vi "step5 TestIfUpperCrossAligned.vi"(8 "error in (no error)":errorcluster, 11 "cube in":T1) -> (0 "error out":errorcluster, 2 "upper cross aligned?":bool)   [LabVIEW 2011]
uses:
  Typedef/cube.ctl
  Typedef/face.ctl
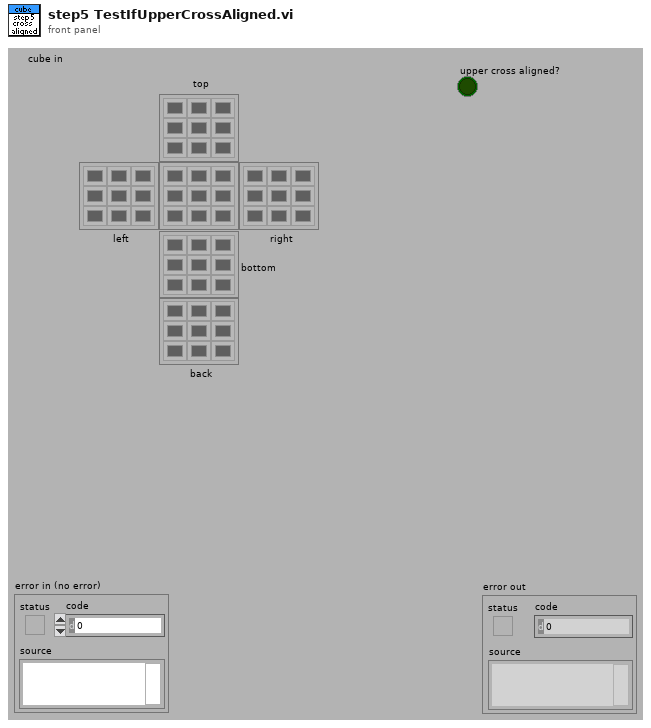
[diagram p1: front panel]
types:
  T1 = typedef "cube.ctl" = cluster{"top":T2, "left":T2, "right":T2, "bottom":T2, "back":T2, "front":T2}
  T2 = typedef "face.ctl" = u32[][]
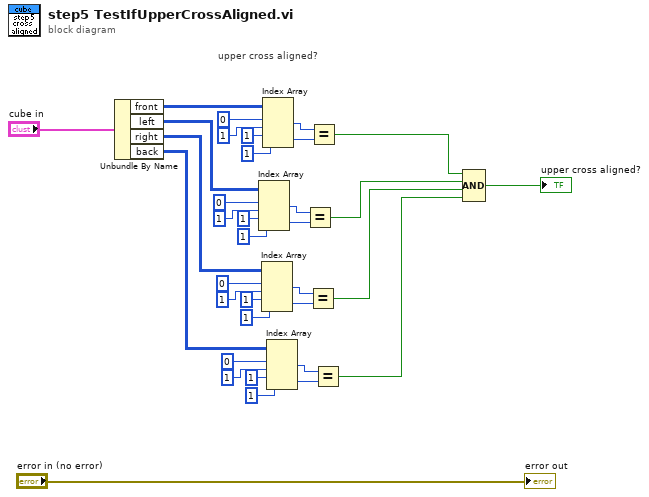
[diagram p0: block diagram]
diagram:
  # "upper cross aligned?"
  n1 = Unbundle By Name("cube in") -> ("front"=w31:T2, "left"=w18:T2, "right"=w11:T2, "back"=w4:T2)
  n2 = Index Array(array=w18, index (row) #1=0 ("index (row)"), index (col) #1=1 ("disabled index (col)"), index (row) #2=1 ("index (row)"), index (col) #2=1 ("disabled index (col)")) -> (element #1=w23:u32, element #2=w24:u32)
  n3 = Index Array(array=w11, index (row) #1=0 ("index (row)"), index (col) #1=1 ("disabled index (col)"), index (row) #2=1 ("index (row)"), index (col) #2=1 ("disabled index (col)")) -> (element #1=w13:u32, element #2=w12:u32)
  n4 = Index Array(array=w31, index (row) #1=0 ("index (row)"), index (col) #1=1 ("disabled index (col)"), index (row) #2=1 ("index (row)"), index (col) #2=1 ("disabled index (col)")) -> (element #1=w26:u32, element #2=w25:u32)
  n5 = Index Array(array=w4, index (row) #1=0 ("index (row)"), index (col) #1=1 ("disabled index (col)"), index (row) #2=1 ("index (row)"), index (col) #2=1 ("disabled index (col)")) -> (element #1=w9:u32, element #2=w10:u32)
  n6 = Equal?(x=w23, y=w24) -> (x = y?=w3:bool)
  n7 = Equal?(x=w13, y=w12) -> (x = y?=w2:bool)
  n8 = Equal?(x=w26, y=w25) -> (x = y?=w33:bool)
  n9 = Equal?(x=w9, y=w10) -> (x = y?=w1:bool)
  n10 = Compound Arithmetic op=AND(w33, w3, w2, w1) -> (→"upper cross aligned?":bool)
  "error out" <- "error in (no error)"
